vi "Create DataBindings.vi"(8 "error in (no error)":errorcluster caption="错误输入（无错误）", 9 "DataMember":string, 10 "dataSource":refnum<k24>, 11 "DataGridView":refnum<k24>) -> (0 "error out":errorcluster caption="错误输出", 3 "DataGridView Out":refnum<k24>)   [LabVIEW 2012, in "DataGridView.lvlib"]
uses:
  DataGridView.lvlib
  System.Windows.Forms
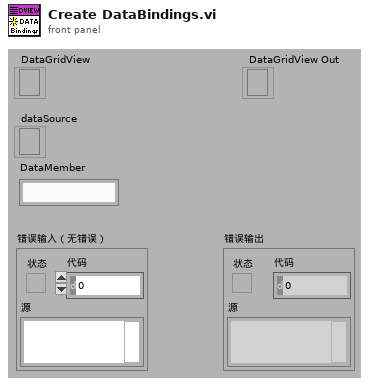
[diagram p1: front panel]
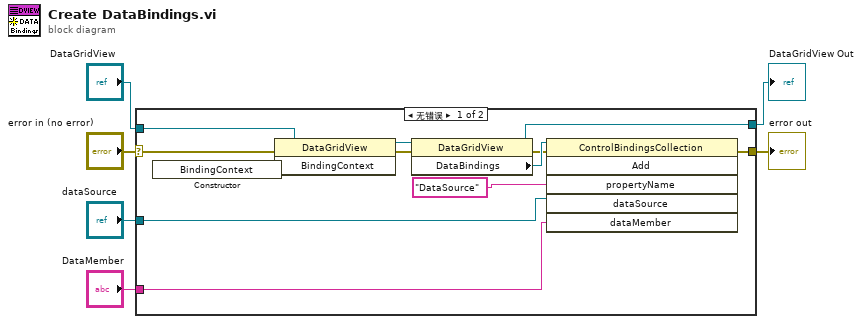
[diagram p0: block diagram]
diagram:
  n1 = case shown="无错误" "error in (no error)" {
    selector: "error in (no error)" -> [w9 w19]
    tunnel: [w10 w19] -> w4
    tunnel: "DataGridView" -> [w18 _]
    tunnel: "DataMember" -> [w12 _]
    tunnel: "dataSource" -> [w8 _]
    tunnel: [w7 _] -> w1
    frame No Error {
      n2 = constructor class="BindingContext"() -> (reference out=w11:refnum<k24>)  [unwired: 3 in, 2 out]
      n3 = property class="DataGridView"(reference=w18, error in=w9, "BindingContext"=w11) -> (reference out=w17:refnum<k24>, error out=w16:errorcluster)
      n4 = property class="DataGridView"(reference=w17, error in=w16) -> (reference out=w7:refnum<k24>, error out=w14:errorcluster, "DataBindings"=w15:refnum<k24>)
      n5 = invoke class="ControlBindingsCollection" method="Add"(reference=w15, error in=w14, "propertyName"="DataSource", "dataSource"=w8, "dataMember"=w12) -> (error out=w10:errorcluster)  [unwired: 1 in, 5 out]
    }
    frame Error {
    }
  }
  "error out" <- w4
  "DataGridView Out" <- w1
